vi "Filter Get Data Averaging Mode.vi"(8 "error in (no error)":errorcluster, 11 "mode":i32) -> (0 "error out":errorcluster, 2 "function return":u32, 3 "mode out":i32)   [LabVIEW 2014, in "atmcd32d.lvlib"]
doc: "unsigned int WINAPI Filter_GetDataAveragingMode(int * mode);"
uses:
  atmcd32d.lvlib
  atmcd32d.dll
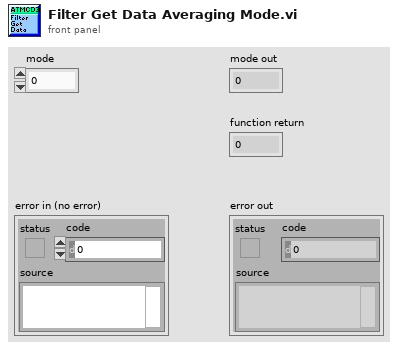
[diagram p1: front panel]
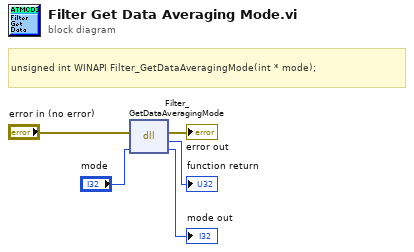
[diagram p0: block diagram]
diagram:
  # "unsigned int WINAPI Filter_GetDataAveragingMode(int * mode);"
  n1 = dll-call lib="C:/Users/Bakir/Documents/Lambda2-Testing/lib/Andorlib/atmcd32d.*" fn="Filter_GetDataAveragingMode"(error in="error in (no error)", "mode"="mode") -> (error out=→"error out":errorcluster, →"function return":u32, "mode"=→"mode out":i32)  [unwired: 2 in, 1 out]
